vi "mag-field_configure.vi"(10 "mag field params in":T1={"mag field"={"from"=0.0, "to"=0.0, "type"=enum."static"}, "use perm mode"=FALSE, "field info out"={"B field (consigne)"=0.0, "B field"=0.0, "B-field driver (vi reference)"=refnum, "consigne ctrl (driver)"=refnum, "field has arrived (ctrl, driver)"=refnum, "field  (ctrl, driver)"=refnum, "Coil supply"=refnum, "GPIB adress"=refnum}, "GPIB adr"="0:1", "driver running?"=FALSE, "ON?"=FALSE, "Coil_Information"={"Max Field 10V Input"=0.0, "Waiting time for 0.5mT step"=0.0, "Dac_Output_Channel"=""}}) -> (2 "mag field params out":T1={"mag field"={"from"=0.0, "to"=0.0, "type"=enum."static"}, "use perm mode"=FALSE, "field info out"={"B field (consigne)"=0.0, "B field"=0.0, "B-field driver (vi reference)"=refnum, "consigne ctrl (driver)"=refnum, "field has arrived (ctrl, driver)"=refnum, "field  (ctrl, driver)"=refnum, "Coil supply"=refnum, "GPIB adress"=refnum}, "GPIB adr"="0:1", "driver running?"=TRUE, "ON?"=TRUE, "Coil_Information"={"Max Field 10V Input"=0.0, "Waiting time for 0.5mT step"=0.0, "Dac_Output_Channel"=""}})   [LabVIEW 2010]
uses:
  mag-field-control.ctl
  type defs - instruments/sweep info.ctl
  type defs - instruments/usage.ctl
  field-info.ctl
panel:
  out "active supply":variant
  out "Mag-field ON":bool
  in  "Main":bool
  in  "STOP":bool
  in  "START":bool
  out "Driver path":path=path "C:/Documents and Settings/User/Bureau/FPGA-clean/fpga-clean/host-subVIs/magnetic field/B-field Driver.vi"
  in  "correct field button":bool
  out "Field (T)":dbl
  in  "Actual Field (T)":dbl
  in  "Coil supply":enum32{"BOUHNIK", "KEPCO"}(tab)
  in  "Use BOUHNIK?":bool
  in  "GPIB adr":string="0:1"
  in  "Use KEPCO?":bool
  out "Dac_Output_Channel":tag
  out "Waiting time for 0.5mT step":dbl
  out "Max Field 10V Input":dbl
  out "vi reference":refnum<vi>
  # "If the field written here doesn't match the actual field, please\nprovide the actual field in the \"Actual Field\" text box and press \"Correct Field\"."
  # "Please check the 120A / 12A switch on the front panel of the power supply.\nThe correct value should be hard wired in \"set-B-field.vi\" prior to running the program"
  # "Note also that use of permanent mode needs the shunt to be off on the\nfront panel of the power supply. You should set the shunt current value though."
  # "The ramp are set in software (close from max ramp speeds). As a consequence, please\nset the ramps at 0 and 0 on the power supply."
  # "In order to be run remotely, the power supply should be started, in 120A or 12A mode (according to what's hard wired in REMOTE INTERFACE)"
  # "The PAC2's extern control has to be wired to the AO 0\nThe current range as to be +/-20A\n\nSet for coil : 0.1453T/A\nMAX : 2.906 T \nMIN : 0 T"
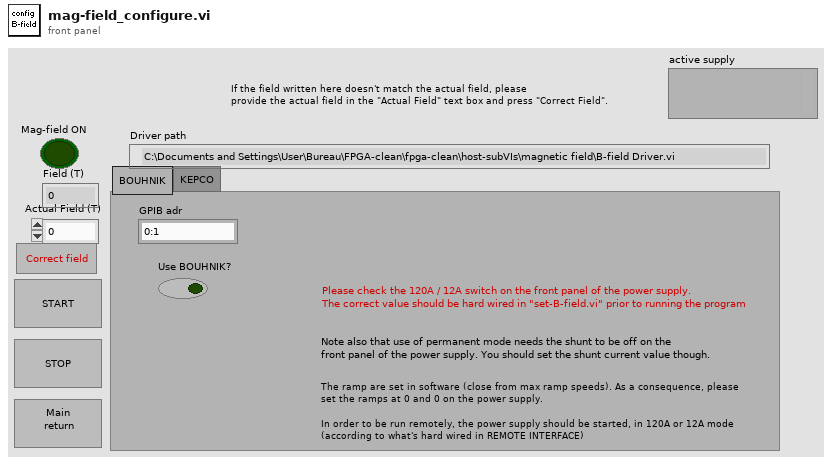
[diagram p1: front panel]
types:
  T1 = typedef "mag-field-control.ctl" = cluster{"mag field":T2, "use perm mode":bool, "field info out":T4, "GPIB adr":string, "driver running?":bool, "ON?":bool, "Coil_Information":cluster{"Max Field 10V Input":dbl, "Waiting time for 0.5mT step":dbl, "Dac_Output_Channel":tag}}
  T2 = typedef "sweep info.ctl" = cluster{"from":sgl, "to":sgl, "type":T3}
  T3 = typedef "usage.ctl" = enum8{"static", "sweep", "step", "step 2", "step 3"}
  T4 = typedef "field-info.ctl" = cluster{"B field (consigne)":dbl, "B field":dbl, "B-field driver (vi reference)":refnum<vi>, "consigne ctrl (driver)":refnum<vi>, "field has arrived (ctrl, driver)":refnum<vi>, "field  (ctrl, driver)":refnum<vi>, "Coil supply":refnum<vi>, "GPIB adress":refnum<vi>}
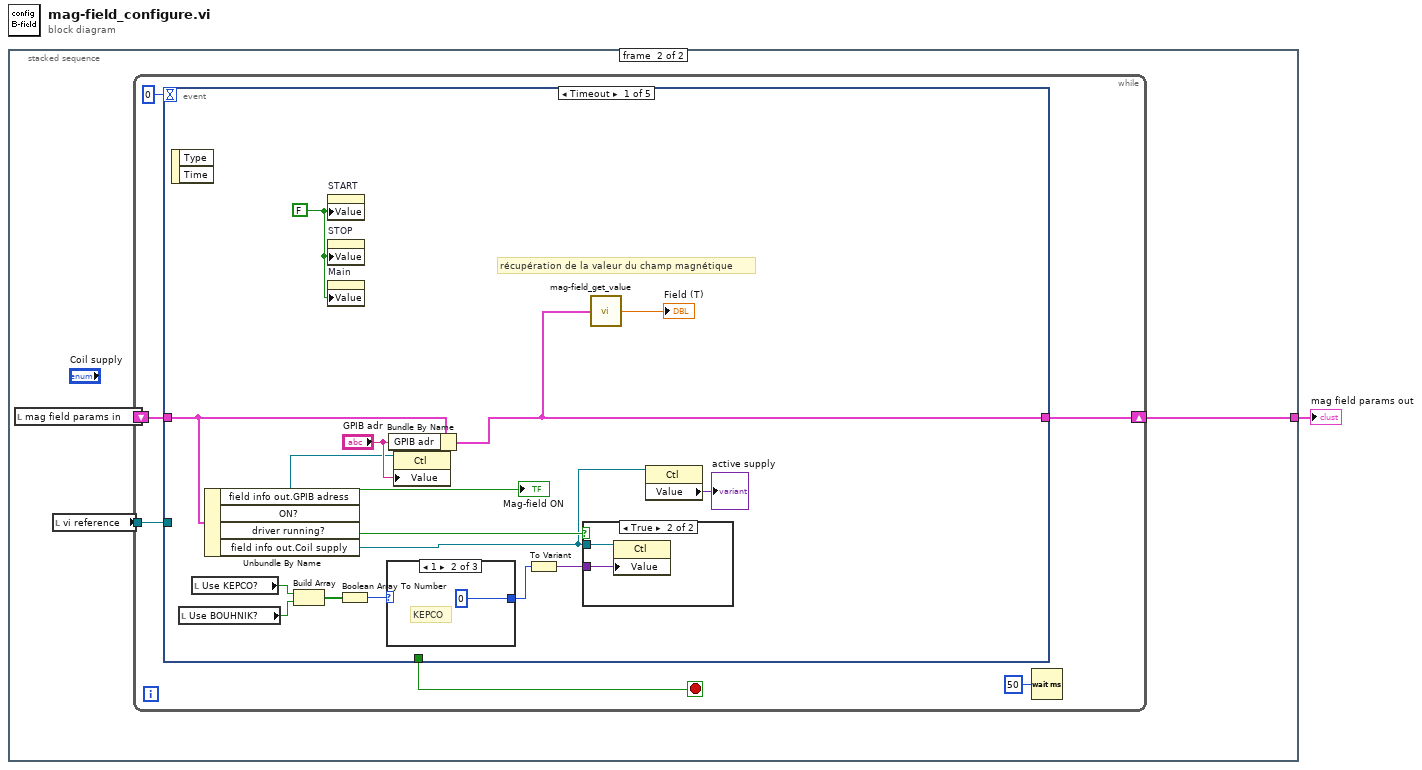
[diagram p0: block diagram]
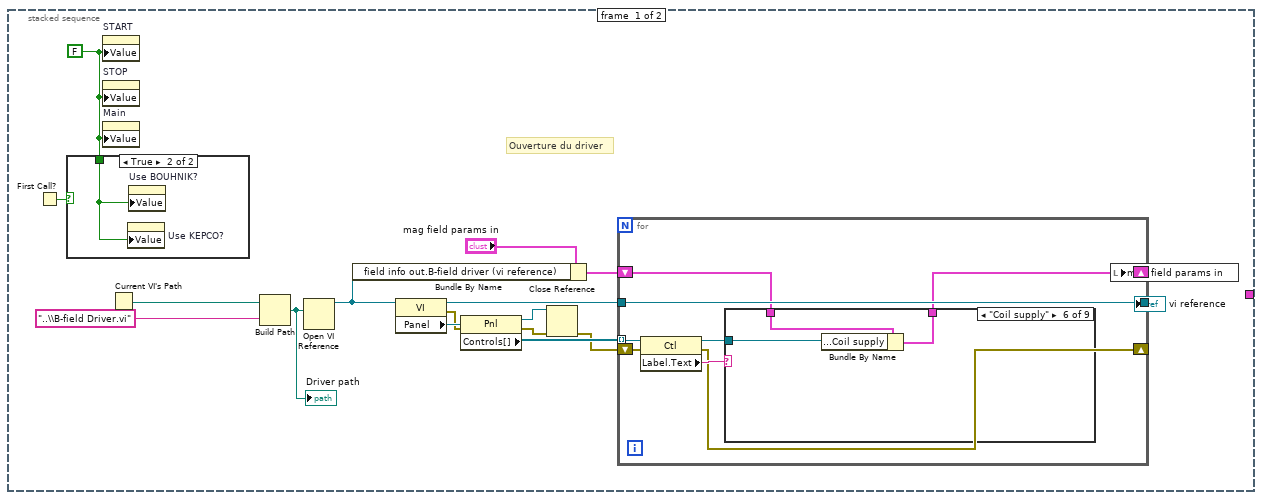
[diagram p2: hidden frame]
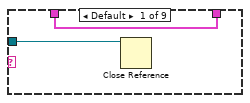
[diagram p4: hidden frame]
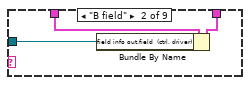
[diagram p5: hidden frame]
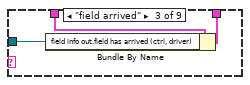
[diagram p6: hidden frame]
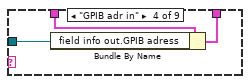
[diagram p7: hidden frame]
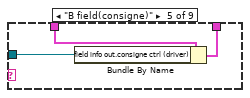
[diagram p8: hidden frame]
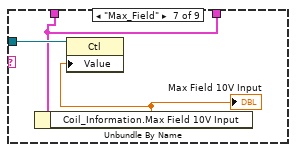
[diagram p9: hidden frame]
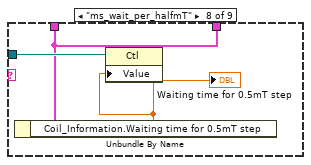
[diagram p10: hidden frame]
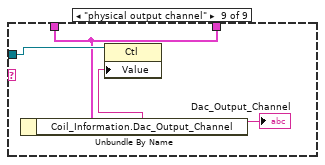
[diagram p11: hidden frame]
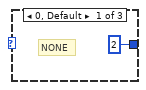
[diagram p13: hidden frame]
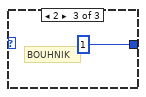
[diagram p14: hidden frame]
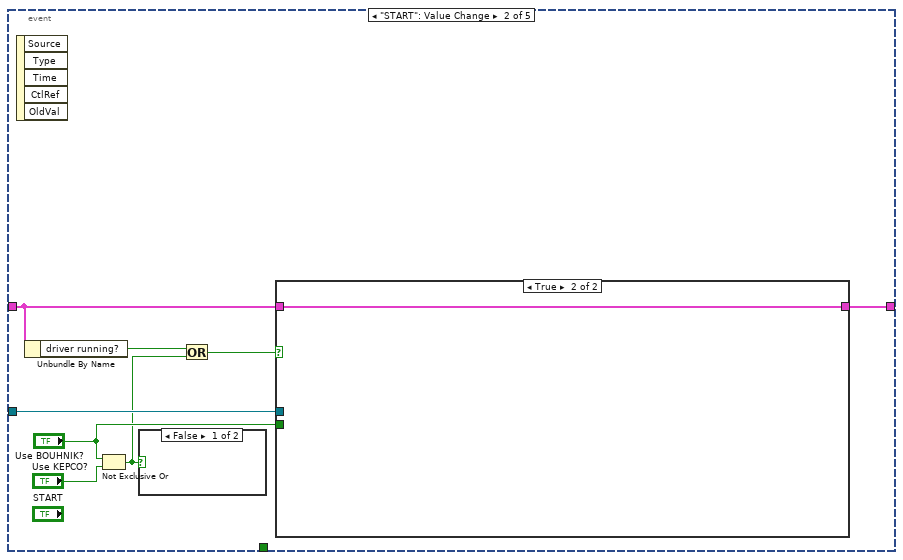
[diagram p15: hidden frame]
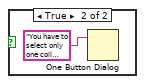
[diagram p16: hidden frame]
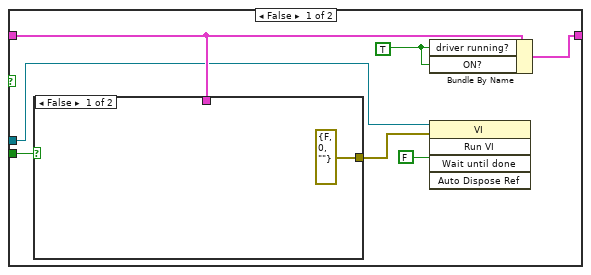
[diagram p17: hidden frame]
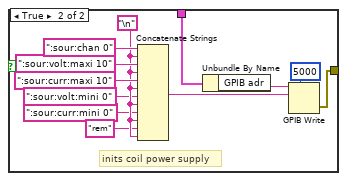
[diagram p18: hidden frame]
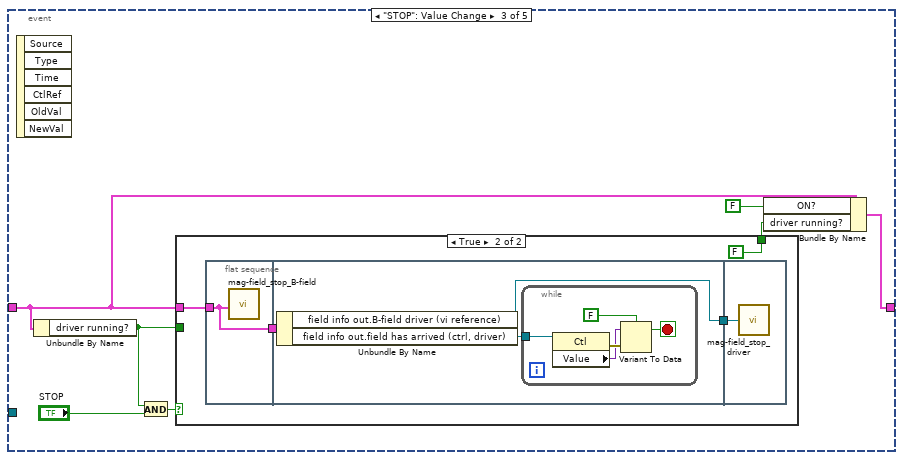
[diagram p19: hidden frame]
diagram:
  n1 = stacked-sequence {
    tunnel: [_ w54] -> w1
    frame #0 {
      w4 = FALSE ("OK Button")
      # "Ouverture du driver"
      n2 = First Call?() -> (First Call?: T/F=w5:bool)
      n3 = case shown="True" w5 {
        tunnel: w4 -> [_ w19]
        frame False {
        }
        frame True {
          n4 = property on="Use KEPCO?" class="Bool (strict)"("Value"=w19) -> ()  [unwired: 2 in, 2 out]
          n5 = property on="Use BOUHNIK?" class="Bool (strict)"("Value"=w19) -> ()  [unwired: 2 in, 2 out]
        }
      }
      n6 = property on="START" class="Bool (strict)"("Value"=w4) -> ()  [unwired: 2 in, 2 out]
      n7 = property on="STOP" class="Bool (strict)"("Value"=w4) -> ()  [unwired: 2 in, 2 out]
      n8 = property on="Main" class="Bool (strict)"("Value"=w4) -> ()  [unwired: 2 in, 2 out]
      n9 = Current VI's Path() -> (path=w8:path)
      n10 = Build Path(base path=w8, name or relative path="..\\B-field Driver.vi") -> (appended path=w10:path)
      "Driver path" <- w10
      n11 = Open VI Reference(vi path=w10) -> (vi reference=w2:refnum<vi>)  [unwired: 2 in, 4 out]
      n12 = Bundle By Name(cluster="mag field params in", "field info out.B-field driver (vi reference)"=w2) -> (w15:T1)
      n13 = property class="VI"(reference=w2) -> (reference out=w16:refnum<vi>, error out=w12:errorcluster, "Panel"=w18:refnum<vi>)  [unwired: 1 in]
      n14 = property class="Pnl"(reference=w18, error in=w12) -> (reference out=w14:refnum<vi>, error out=w13:errorcluster, "Controls[]"=w17:refnum<vi>[])
      n15 = Close Reference(reference=w14, error in (no error)=w13) -> (error out=w11:errorcluster)
      n16 = for {
        tunnel: w17 -> [w27] mode=indexing
        tunnel: [w24] -> w9
        tunnel: w16 -> [w24]
        shift-right: [w22] -> w6
        shift-left: w15 -> [w23]
        shift-right: [w20] -> _
        shift-left: w11 -> [w21]
        n17 = property class="Ctl"(reference=w27, error in=w21) -> (reference out=w25:refnum<vi>, error out=w20:errorcluster, "Label.Text"=w26:string)
        n18 = case shown="\"Coil supply\"" w26 {
          tunnel: w25 -> [w28 w30 w33 w36 w40 w42 w47 w50 w53]
          tunnel: w23 -> [w29 w32 w35 w38 w41 w44 w45 w48 w52]
          tunnel: [w29 w31 w34 w37 w39 w43 w45 w48 w52] -> w22
          frame Default {
            n19 = Close Reference(reference=w28) -> ()  [unwired: 1 in, 1 out]
          }
          frame "B field" {
            n20 = Bundle By Name(cluster=w32, "field info out.field  (ctrl, driver)"=w30) -> (w31:T1)
          }
          frame "field arrived" {
            n21 = Bundle By Name(cluster=w35, "field info out.field has arrived (ctrl, driver)"=w33) -> (w34:T1)
          }
          frame "GPIB adr in" {
            n22 = Bundle By Name(cluster=w38, "field info out.GPIB adress"=w36) -> (w37:T1)
          }
          frame "B field(consigne)" {
            n23 = Bundle By Name(cluster=w41, "field info out.consigne ctrl (driver)"=w40) -> (w39:T1)
          }
          frame "Coil supply" {
            n24 = Bundle By Name(cluster=w44, "field info out.Coil supply"=w42) -> (w43:T1)
          }
          frame "Max_Field" {
            n25 = Unbundle By Name(w45) -> ("Coil_Information.Max Field 10V Input"=w46:dbl)
            "Max Field 10V Input" <- w46
            n26 = property class="Ctl"(reference=w47, "Value"=w46) -> ()  [unwired: 1 in, 2 out]
          }
          frame "ms_wait_per_halfmT" {
            n27 = Unbundle By Name(w48) -> ("Coil_Information.Waiting time for 0.5mT step"=w49:dbl)
            "Waiting time for 0.5mT step" <- w49
            n28 = property class="Ctl"(reference=w50, "Value"=w49) -> ()  [unwired: 1 in, 2 out]
          }
          frame "physical output channel" {
            n29 = Unbundle By Name(w52) -> ("Coil_Information.Dac_Output_Channel"=w51:tag)
            "Dac_Output_Channel" <- w51
            n30 = property class="Ctl"(reference=w53, "Value"=w51) -> ()  [unwired: 1 in, 2 out]
          }
        }
      }
      "vi reference" <- w9
      n31 = local write "mag field params in"(w6) -> ()
    }
    frame #1 {
      n32 = local read "mag field params in"() -> (w55:T1)
      n33 = local read "vi reference"() -> (w56:refnum<vi>)
      n34 = while {
        shift-right: [w60] -> w54
        shift-left: w55 -> [w61]
        tunnel: w56 -> [w59]
        stop <- w62 stop-if-true
        n35 = event shown="[0] Timeout" {
          selector: _ -> [_ _ _ _ _]
          dyn-events: _ -> [_ _ _ _ _]
          timeout: 0 -> [_ _ _ _ _]
          tunnel: [_ _ _ "Main" _] -> w62
          tunnel: w61 -> [w68 w87 w118 w136 w141]
          tunnel: [w65 w90 w116 w136 w140] -> w60
          tunnel: w59 -> [_ w91 _ _ w139]
          event Timeout {
            w70 = FALSE ("OK Button")
            # "récupération de la valeur du champ magnétique"
            n36 = event-data() -> ()  [unwired: 3 out]
            n37 = local read "Use BOUHNIK?"() -> (w75:bool)
            n38 = local read "Use KEPCO?"() -> (w76:bool)
            n39 = Unbundle By Name(w68) -> ("field info out.GPIB adress"=w66:refnum<vi>, "ON?"=→"Mag-field ON":bool, "driver running?"=w71:bool, "field info out.Coil supply"=w64:refnum<vi>)
            n40 = Build Array(w76, w75) -> (w74:bool[])
            n41 = property on="START" class="Bool (strict)"("Value"=w70) -> ()  [unwired: 2 in, 2 out]
            n42 = property on="STOP" class="Bool (strict)"("Value"=w70) -> ()  [unwired: 2 in, 2 out]
            n43 = property on="Main" class="Bool (strict)"("Value"=w70) -> ()  [unwired: 2 in, 2 out]
            n44 = Boolean Array To Number(Boolean array=w74) -> (number=w73:u32)
            n45 = case shown="1" w73 {
              tunnel: [u32 2 u32 0 u32 1] -> w72
              frame 0, Default {
                # "NONE"
              }
              frame 1 {
                # "KEPCO"
              }
              frame 2 {
                # "BOUHNIK"
              }
            }
            n46 = Bundle By Name(cluster=w68, "GPIB adr"="GPIB adr") -> (w65:T1)
            n47 = property class="Ctl"(reference=w66, "Value"="GPIB adr") -> ()  [unwired: 1 in, 2 out]
            n48 = To Variant(anything=w72) -> (Variant=w77:variant)
            n49 = case shown="True" w71 {
              tunnel: w77 -> [_ w80]
              tunnel: w64 -> [_ w79]
              frame False {
              }
              frame True {
                n50 = property class="Ctl"(reference=w79, "Value"=w80) -> ()  [unwired: 1 in, 2 out]
              }
            }
            n51 = call "mag-field_get_value.vi"("mag fiel params"=w65) -> ("field"=→"Field (T)":dbl)
            n52 = property class="Ctl"(reference=w64) -> ("Value"=→"active supply":variant)  [unwired: 1 in, 2 out]
          }
          event "START": Value Change {
            n53 = event-data() -> ()  [unwired: 6 out]
            n54 = Unbundle By Name(w87) -> ("driver running?"=w86:bool)
            n55 = Not Exclusive Or(1:"Use KEPCO?", 2:"Use BOUHNIK?") -> (0:w85:bool)
            n56 = case shown="False" w85 {
              frame False {
              }
              frame True {
                n57 = One Button Dialog(message="You have to select only one coil supply") -> ()  [unwired: 2 out]
              }
            }
            n58 = Or(x=w86, y=w85) -> (x .or. y?=w84:bool)
            n59 = case shown="True" w84 {
              tunnel: w91 -> [w93 _]
              tunnel: w87 -> [w97 w113]
              tunnel: [w98 w113] -> w90
              tunnel: "Use BOUHNIK?" -> [w95 _]
              frame False {
                w94 = TRUE ("driver running?")
                n60 = case shown="False" w95 {
                  tunnel: w97 -> [_ w102]
                  tunnel: [errorcluster {"status"=FALSE, "code"=0, "source"=""} ("error out") w101] -> w96
                  frame False {
                  }
                  frame True {
                    w108 = "\n"
                    # "inits coil power supply"
                    n61 = Concatenate Strings(":sour:chan 0" ("string"), w108, ":sour:volt:maxi 10" ("string"), w108, ":sour:curr:maxi 10" ("string"), w108, ":sour:volt:mini 0" ("string"), w108, ":sour:curr:mini 0" ("string"), w108, "rem" ("string"), w108) -> (w112:string)
                    n62 = Unbundle By Name(w102) -> ("GPIB adr"=w104:string)
                    n63 = GPIB Write(0:w104, 1:w112, 4:5000 ("timeout ms (488.2 global)")) -> (6:w101:errorcluster)  [unwired: 1 in, 2 out]
                  }
                }
                n64 = Bundle By Name(cluster=w97, "driver running?"=w94, "ON?"=w94) -> (w98:T1)
                n65 = invoke class="VI" method="Run VI"(reference=w93, error in=w96, "Wait until done"=FALSE ("Wait Until Done")) -> ()  [unwired: 2 in, 5 out]
              }
              frame True {
              }
            }
          }
          event "STOP": Value Change {
            n66 = event-data() -> ()  [unwired: 7 out]
            n67 = Unbundle By Name(w118) -> ("driver running?"=w114:bool)
            n68 = And(x=w114, y="STOP") -> (x .and. y?=w119:bool)
            n69 = case shown="True" w119 {
              tunnel: w118 -> [_ w125]
              tunnel: [w121 FALSE ("ON?")] -> w115
              tunnel: w114 -> [w121 _]
              frame False {
              }
              frame True {
                n70 = flat-sequence {
                  tunnel: w125 -> [w126]
                  tunnel: [w126] -> w124
                  tunnel: w124 -> [w129]
                  tunnel: [w127] -> w123
                  tunnel: w123 -> [w135]
                  frame #0 {
                    n71 = call "mag-field_stop_B-field.vi"("mag fiel params"=w126) -> ()  [unwired: 11 out]
                  }
                  frame #1 {
                    n72 = Unbundle By Name(w129) -> ("field info out.B-field driver (vi reference)"=w127:refnum<vi>, "field info out.field has arrived (ctrl, driver)"=w128:refnum<vi>)
                    n73 = while {
                      tunnel: w128 -> [w134]
                      stop <- w130 stop-if-true
                      n74 = property class="Ctl"(reference=w134) -> (error out=w133:errorcluster, "Value"=w132:variant)  [unwired: 1 in, 1 out]
                      n75 = Variant To Data(error in=w133, Variant=w132, type=FALSE) -> (data=w130:bool)  [unwired: 1 out]
                    }
                  }
                  frame #2 {
                    n76 = call "mag-field_stop_driver.vi"("B-field driver ref"=w135) -> ()
                  }
                }
              }
            }
            n77 = Bundle By Name(cluster=w118, "ON?"=FALSE, "driver running?"=w115) -> (w116:T1)
          }
          event "Main": Value Change {
            n78 = event-data() -> ()  [unwired: 7 out]
          }
          event "correct field button": Value Change {
            n79 = event-data() -> ()  [unwired: 7 out]
            n80 = case shown="True" "correct field button" {
              selector: "correct field button" -> [w164 _]
              tunnel: [w164 w166] -> w142
              tunnel: "Actual Field (T)" -> [_ w165]
              frame False {
              }
              frame True {
                n81 = Number To Exponential String(number=w165) -> (E-format string=w168:string)  [unwired: 3 out]
                n82 = Concatenate Strings("Are you sure the actual field is:\n" ("message"), w168, " T\n\nand you want to proceed with this value?" ("string")) -> (w169:string)
                n83 = Two Button Dialog(message=w169) -> (T button?=w166:bool)  [unwired: 2 out]
              }
            }
            n84 = case shown="True" w142 {
              tunnel: "Actual Field (T)" -> [_ w148]
              tunnel: w141 -> [w144 w150]
              tunnel: [w144 w150] -> w140
              tunnel: w139 -> [_ w149]
              frame False {
              }
              frame True {
                n85 = flat-sequence {
                  tunnel: w149 -> [w153]
                  tunnel: w150 -> [w154]
                  tunnel: [w154] -> w147
                  tunnel: [w152] -> w146
                  tunnel: [w151] -> w145
                  tunnel: w148 -> [w157]
                  tunnel: w147 -> [w163]
                  tunnel: w146 -> [w160]
                  tunnel: w145 -> [w156]
                  frame #0 {
                    n86 = invoke class="VI" method="Abort VI"(reference=w153) -> (reference out=w152:refnum<vi>, error out=w151:errorcluster)  [unwired: 2 in, 1 out]
                  }
                  frame #1 {
                    n87 = Unbundle By Name(w163) -> ("field info out.field  (ctrl, driver)"=w162:refnum<vi>, "field info out.consigne ctrl (driver)"=w155:refnum<vi>)
                    n88 = property class="Ctl"(reference=w162, error in=w156, "Value"=w157) -> (error out=w159:errorcluster)  [unwired: 1 out]
                    n89 = property class="Ctl"(reference=w155, error in=w159, "Value"=w157) -> (error out=w158:errorcluster)  [unwired: 1 out]
                    n90 = invoke class="VI" method="Run VI"(reference=w160, error in=w158, "Wait until done"=FALSE ("Wait Until Done")) -> ()  [unwired: 2 in, 5 out]
                  }
                }
              }
            }
          }
        }
        n91 = Wait (ms)(milliseconds to wait=u32 50) -> ()  [unwired: 1 out]
      }
    }
  }
  "mag field params out" <- w1
